vi "Measurement Logic.vi"() -> ()   [LabVIEW 2021, in "DmmMeasurementHAL.lvlib"]
uses:
  DmmMeasurementHAL.lvlib
  Measurement Configuration.ctl
  Measurement Results.ctl
  <vilib>/Plug-In SDKs/Measurements/Measure Call Context/Measure Call Context.lvclass
  <vilib>/Plug-In SDKs/Clients/Session Management V1/Session Reservation/Initialize and Close Session Behavior.ctl
  HAL/Instruments/DMM_Base/Utility/Get 1 Pin Object.vi
  HAL/Instruments/DMM_Base/DMM_Base.lvclass
  <vilib>/Plug-In SDKs/Clients/Session Management V1/Session Reservation/Session Reservation.lvclass
panel:
  out "measure call context out":refnum<class "Measure Call Context.lvclass">
  in  "measure call context in":refnum<class "Measure Call Context.lvclass">
  out "measurement results":T1 {"Measurement" format="%.6p"}
  in  "measurement configuration":T2={"pin_name"="Lorem ipsum dolor sit", "Range"=1.2, "Measurement Type"=enum."DC Volts", "Resolution in Digits"=enum."3 1/2"}
  out "error out":errorcluster
  in  "error in":errorcluster
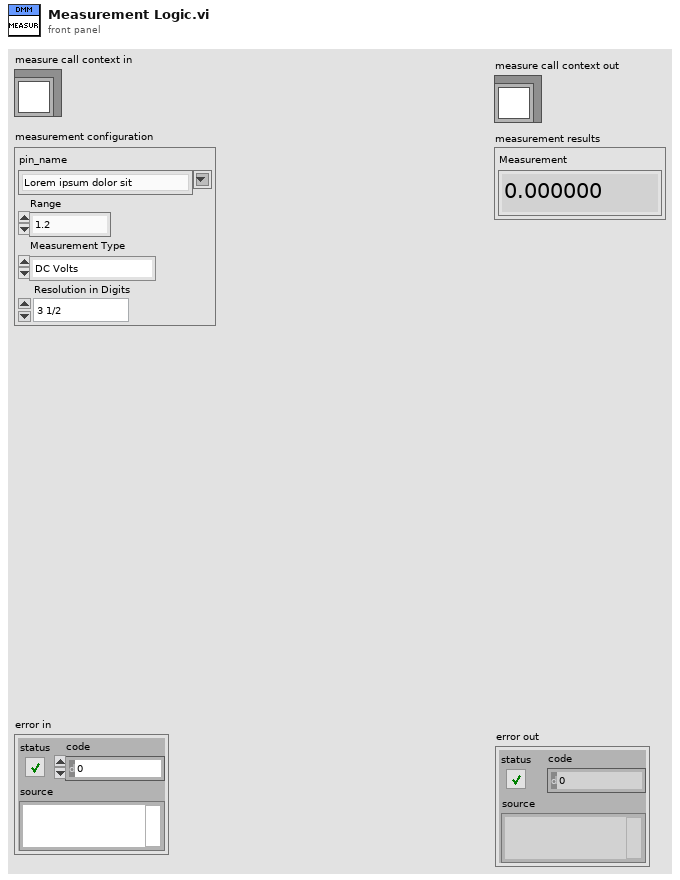
[diagram p1: front panel]
types:
  T1 = typedef "DmmMeasurementHAL.lvlib/Measurement Results.ctl" = cluster{"Measurement":dbl}
  T2 = typedef "DmmMeasurementHAL.lvlib/Measurement Configuration.ctl" = cluster{"pin_name":string, "Range":dbl, "Measurement Type":enum32{"DC Volts", "AC Volts", "DC Current", "AC Current", "2-wire Resistance", "4-wire Resistance", "Diode", "Frequency", "Period", "AC Volts DC Coupled", "Capacitance", "Inductance", "Temperature"}, "Resolution in Digits":enum32{"3 1/2", "4 1/2", "5 1/2", "6 1/2", "7 1/2"}}
  T3 = typedef "NI Session Management V1 Client.lvlib/Session Reservation.lvclass/Initialize and Close Session Behavior.ctl" = enum16{"Auto", "Initialize and Close", "Attach and Detach", "Initialize and Detach", "Attach and Close"}
  T4 = enum32{"3 1/2", "4 1/2", "5 1/2", "6 1/2", "7 1/2"}
  T5 = enum32{"DC Volts", "AC Volts", "DC Current", "AC Current", "2-wire Resistance", "4-wire Resistance", "Diode", "Frequency", "Period", "AC Volts DC Coupled", "Capacitance", "Inductance", "Temperature"}
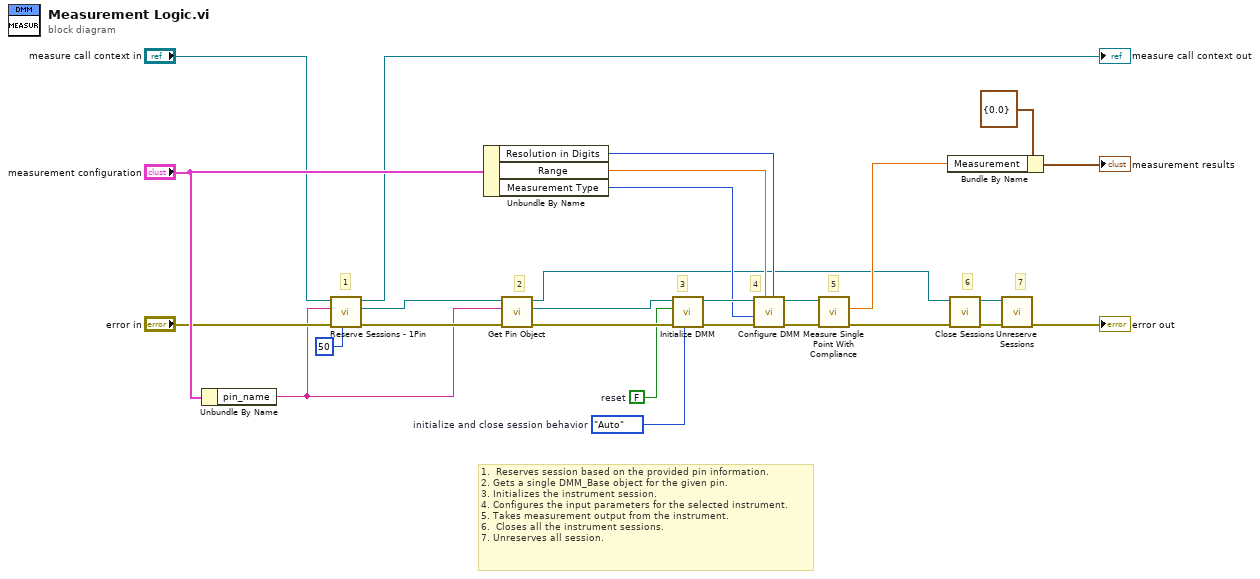
[diagram p0: block diagram]
diagram:
  w3 = Initialize_and_Close_Session_Behavior."Auto"  # initialize and close session behavior
  w4 = FALSE  # reset
  # "1.  Reserves session based on the provided pin information.\n2. Gets a single DMM_Base object for the given pin.\n3. Initializes the instrument session.\n4. Configures the input parameters for the selected instrument.\n5. Takes measurement output from the instrument.\n6.  Closes all the instrument sessions.\n7. Unreserves all session."
  # "7"
  # "6"
  # "5"
  # "4"
  # "3"
  # "2"
  # "1"
  n1 = Unbundle By Name("measurement configuration") -> ("pin_name"=w6:string)
  n2 = call <vilib>:"Reserve Sessions - 1Pin.vi"("timeout (ms)"=50, "error in"="error in", "pin or relay name"=w6, "measurement context in"="measure call context in") -> ("error out"=w10:errorcluster, "session reservation out"=w7:refnum<class "Session Reservation.lvclass">, "measurement context out"=→"measure call context out":refnum<class "Measure Call Context.lvclass">)  [unwired: 5 in]
  n3 = Unbundle By Name("measurement configuration") -> ("Resolution in Digits"=w23:T4, "Range"=w22:dbl, "Measurement Type"=w21:T5)
  n4 = call-poly "Get Pin Object.vi"("error in"=w10, "pin or relay name"=w6, "session reservation in"=w7) -> ("error out"=w12:errorcluster, "instrument object"=w1:refnum<class "DMM_Base.lvclass">, "session reservation out"=w5:refnum<class "Session Reservation.lvclass">)  [unwired: 6 in]
  n5 = call-dynamic "Initialize DMM.vi"("initialize and close session behavior"=w3, "error in (no error)"=w12, "reset"=w4, "DMM_Base in"=w1) -> ("error out"=w27:errorcluster, "DMM_Base out"=w25:refnum<class "DMM_Base.lvclass">)  [unwired: 6 in]
  n6 = call-dynamic "Configure DMM.vi"("Resolution in Digits"=w23, "Range"=w22, "error in (no error)"=w27, "Measurement Type"=w21, "DMM_Base in"=w25) -> ("error out"=w26:errorcluster, "DMM_Base out"=w20:refnum<class "DMM_Base.lvclass">)  [unwired: 5 in]
  n7 = call-dynamic "Measure Single Point With Compliance.vi"("error in (no error)"=w26, "DMM_Base in"=w20) -> ("error out"=w15:errorcluster, "Measured_Value"=w18:dbl)  [unwired: 6 in, 2 out]
  n8 = Bundle By Name(cluster=T1 {"Measurement"=0.0} ("measurement results"), "Measurement"=w18) -> (→"measurement results":T1)
  n9 = call <vilib>:"Close Sessions.vi"("error in"=w15, "session reservation in"=w5) -> ("error out"=w16:errorcluster, "session reservation out"=w13:refnum<class "Session Reservation.lvclass">)  [unwired: 8 in]
  n10 = call <vilib>:"Unreserve Sessions.vi"("error in"=w16, "session reservation in"=w13) -> ("error out"=→"error out":errorcluster)  [unwired: 9 in]
